vi "VelocityControl.vi"(0 "estimatives":T5, 1 "Dest_orientation":dbl, 2 "Position":dbl[](array[numeric]), 3 "Waypoint 1":dbl[](array[numeric]), 4 "Waypoint 0":dbl[](array[numeric]), 5 "Vx":dbl format="%#_13g", 7 "Project":T2, 9 "Vy":dbl format="%#_13g", 10 "VSSStates":T1, 11 "output xy":dbl=2.4, 12 "output inc":dbl=2.4, 13 "output angle":dbl=4.0, 14 "PID gains Vel":T4={"proportional gain (Kc)"=0.6, "integral time (Ti, min)"=0.0, "derivative time (Td, min)"=0.0}, 15 "Path  Smooth":dbl[][](array[numeric])) -> (8 "Output Velocity":dbl[](array[numeric]) format="%.2f")   [LabVIEW 2023]
uses:
  Controle/VelocityGraph.ctl
  Parameters_class/Project.ctl
  VSSNavigation/VSSAttackerStates.ctl
  <vilib>/Analysis/coordinate.llb/Wrap Angle (scalar).vi
  <vilib>/Analysis/coordinate.llb/2D Cartesian Coordinate Rotation (Scalar).vi
  <vilib>/Analysis/NI_AAL_Angle.lvlib
  <vilib>/Analysis/NI_AALPro.lvlib
panel:
  out "Velocity Y":T3
  out "Velocity X":T3
  in  "PID Gains Angle":T4={"proportional gain (Kc)"=5.0, "integral time (Ti, min)"=0.0, "derivative time (Td, min)"=-2.0}
  in  "Reinitialize":bool
  in  "PID Gains lateral":T4={"proportional gain (Kc)"=0.1, "integral time (Ti, min)"=0.0, "derivative time (Td, min)"=0.0}
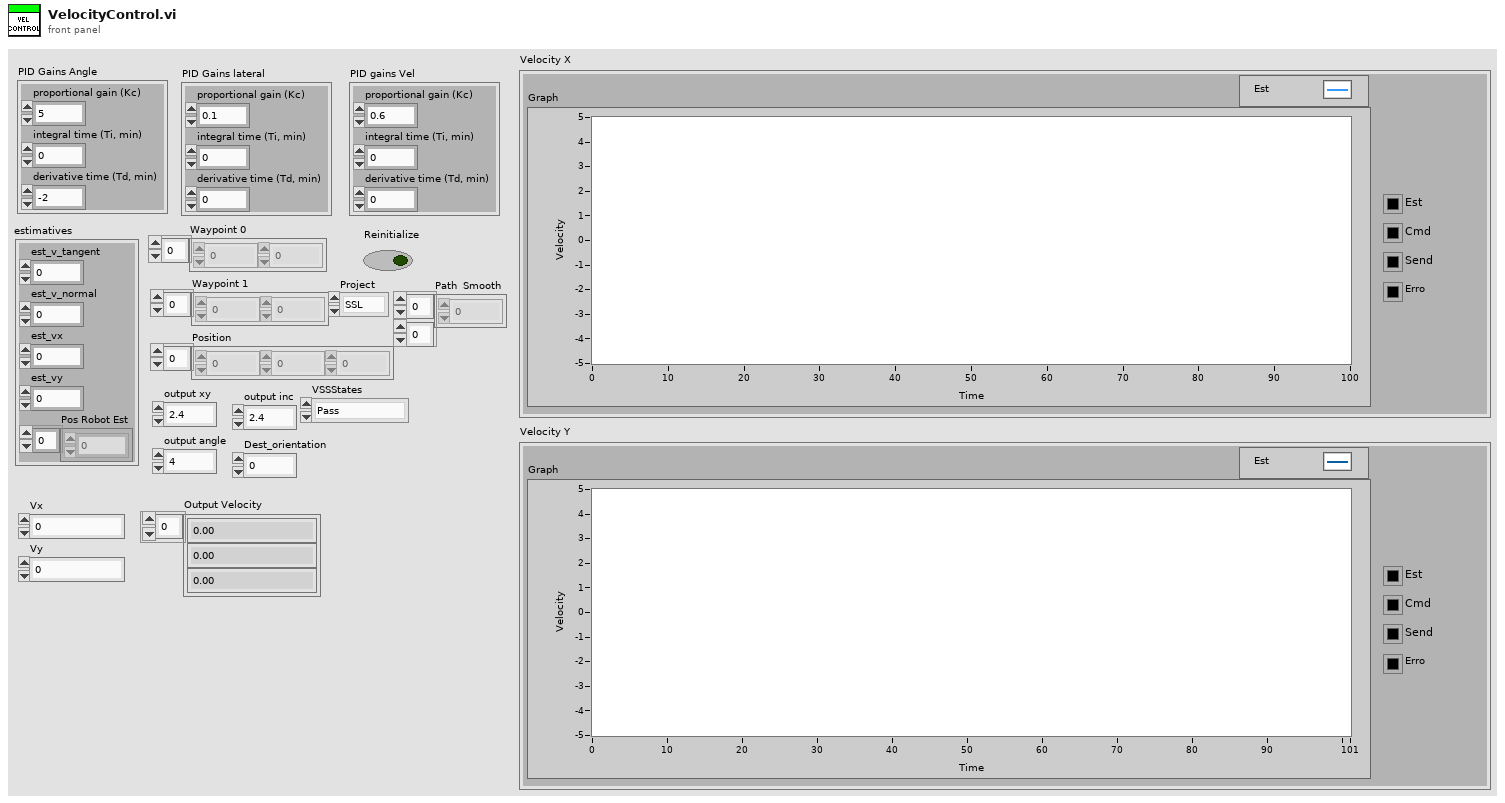
[diagram p1: front panel]
types:
  T1 = typedef "VSSAttackerStates.ctl" = enum16{"Pass", "GoToTangent", "BallGetting", "GoToKick", "Rotate anti-clockwise", "Rotate Clockwise", ""}
  T2 = typedef "Project.ctl" = enum16{"SSL", "VSS"}
  T3 = typedef "VelocityGraph.ctl" = cluster{"Graph":cluster{"est_vx":dbl, "Vx":dbl, dbl, "x out":dbl}, "Est":u32, "Cmd":u32, "Send":u32, "Erro":u32}
  T4 = cluster{"proportional gain (Kc)":dbl, "integral time (Ti, min)":dbl, "derivative time (Td, min)":dbl}
  T5 = cluster{"est_v_tangent":dbl, "est_v_normal":dbl, "est_vx":dbl, "est_vy":dbl, "Pos Robot Est":dbl[]}
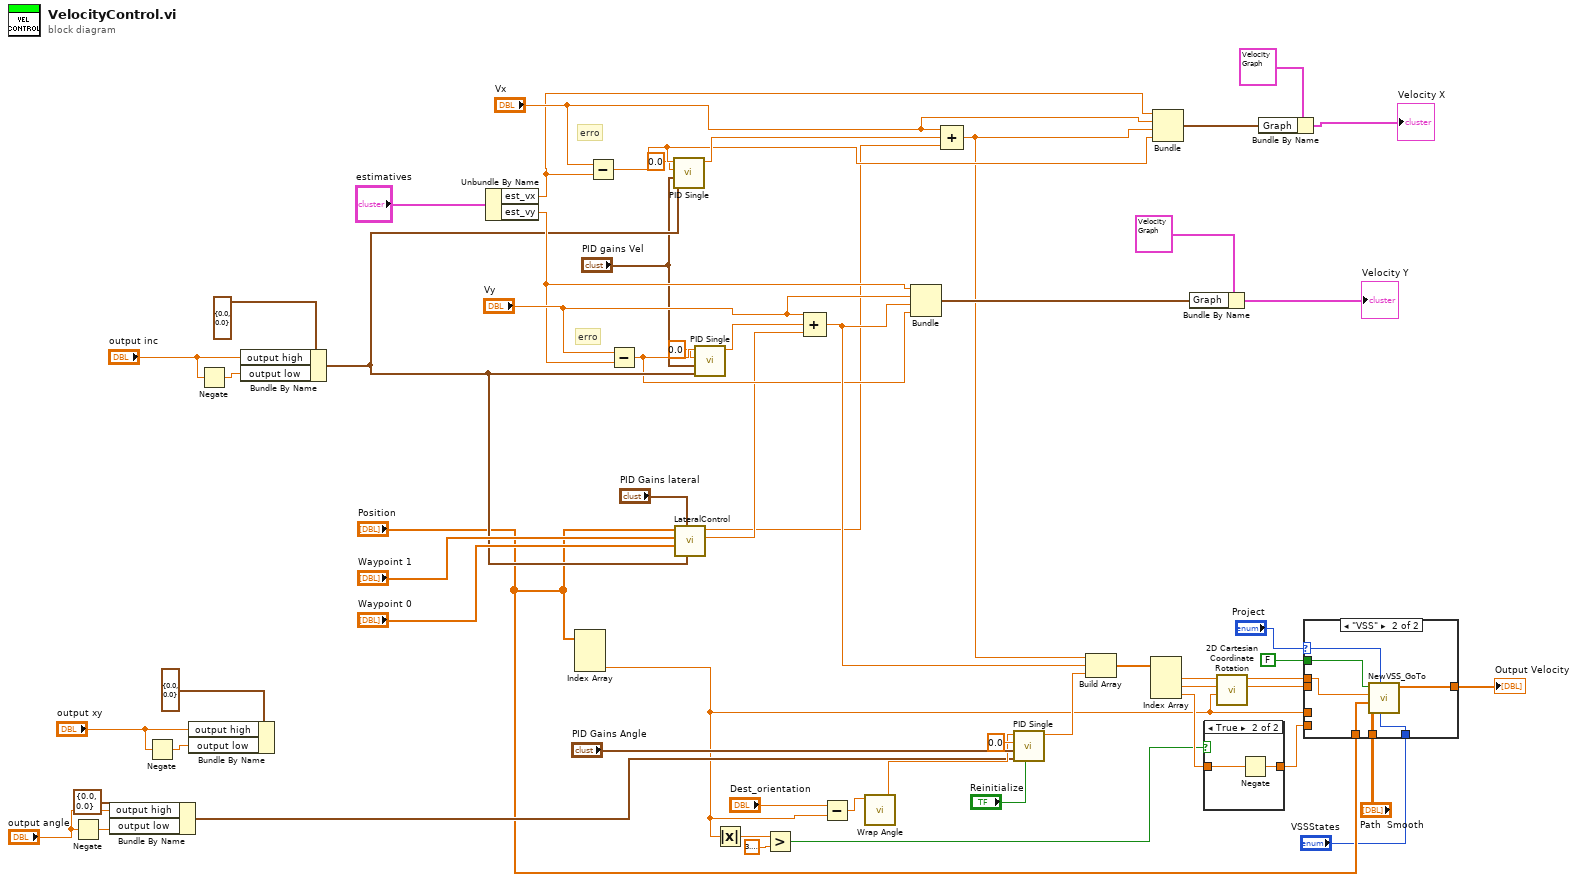
[diagram p0: block diagram]
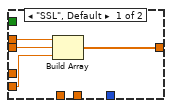
[diagram p2: hidden frame]
diagram:
  # "erro"
  # "erro"
  n1 = Negate(x="output angle") -> (-x=w43:dbl)
  n2 = Bundle By Name(cluster=cluster{"output high":dbl, "output low":dbl} {"output high"=0.0, "output low"=0.0}, "output high"="output angle", "output low"=w43) -> (w18:cluster{"output high":dbl, "output low":dbl})
  n3 = Negate(x="output xy") -> (-x=w45:dbl)
  n4 = Bundle By Name(cluster=cluster{"output high":dbl, "output low":dbl} {"output high"=0.0, "output low"=0.0} ("new element/subarray"), "output high"="output xy", "output low"=w45) -> ()  [unwired: 1 out]
  n5 = Negate(x="output inc") -> (-x=w28:dbl)
  n6 = Bundle By Name(cluster=cluster{"output high":dbl, "output low":dbl} {"output high"=0.0, "output low"=0.0} ("new element/subarray"), "output high"="output inc", "output low"=w28) -> (w17:cluster{"output high":dbl, "output low":dbl})
  n7 = Unbundle By Name("estimatives") -> ("est_vx"=w26:dbl, "est_vy"=w25:dbl)
  n8 = Index Array(array="Position") -> (element #3=w6:dbl)  [unwired: 3 in, 2 out]
  n9 = Subtract(x="Vx", y=w26) -> (x-y=w16:dbl)
  n10 = Subtract(x="Vy", y=w25) -> (x-y=w14:dbl)
  n11 = call "PID Single.vi"("Limits"=w17, "PID gains in"="PID gains Vel", "Variable"=0.0 ("Setpoint"), "Setpoint"=w16) -> ("Out"=w34:dbl)  [unwired: 7 in]
  n12 = call "LateralControl.vi"("output range"=w17, "PID Gains lateral"="PID Gains lateral", "Waypoint 0"="Waypoint 0", "Waypoint 1"="Waypoint 1", "Position"="Position") -> ("y out"=w11:dbl, "x out"=w10:dbl)  [unwired: 5 in]
  n13 = call "PID Single.vi"("Limits"=w17, "PID gains in"="PID gains Vel", "Variable"=0.0 ("Setpoint"), "Setpoint"=w14) -> ("Out"=w33:dbl)  [unwired: 7 in]
  n14 = Absolute Value(x=w6) -> (abs(x)=w57:dbl)
  n15 = Greater?(x=w57, y=3.141592653589793) -> (0:w52:bool)
  n16 = Compound Arithmetic op=ADD("Vy", w33, w11) -> (w30:dbl)
  n17 = Subtract(x="Dest_orientation", y=w6) -> (x-y=w49:dbl)
  n18 = call-poly <vilib>:"Wrap Angle.vi"("angle in"=w49) -> ("angle out"=w48:dbl)  [unwired: 9 in, 1 out]
  n19 = Bundle("est_vy"=w25, "Vy"="Vy", w30, w14) -> (w23:cluster{"est_vy":dbl, "Vy":dbl, dbl, dbl})  [unwired: 1 in]
  n20 = Compound Arithmetic op=ADD("Vx", w34, w10) -> (w9:dbl)
  n21 = call "PID Single.vi"("initialize"="Reinitialize", "Limits"=w18, "PID gains in"="PID Gains Angle", "Variable"=0.0, "Setpoint"=w48) -> ("Out"=w53:dbl)  [unwired: 6 in]
  n22 = Build Array(w9, w30, w53) -> (w7:dbl[])
  n23 = Index Array(array=w7) -> (element #1=w8:dbl, element #2=w60:dbl, element #3=w56:dbl)  [unwired: 3 in]
  n24 = Bundle("est_vx"=w26, "Vx"="Vx", w9, w16) -> (w20:cluster{"est_vx":dbl, "Vx":dbl, dbl, dbl})  [unwired: 1 in]
  n25 = Bundle By Name(cluster=T3 {"Graph"={"est_vx"=-0.14571416207204627, "Vx"=0.4692407651588243, 1.5797768746041183, "x out"=1.110536109445294}, "Est"=16860, "Cmd"=16711680, "Send"=6618880, "Erro"=16776722} ("Velocity Y"), "Graph"=w23) -> (→"Velocity Y":T3)
  n26 = case shown="True" w52 {
    tunnel: w56 -> [w61 w63]
    tunnel: [w61 w62] -> w55
    frame False {
    }
    frame True {
      n27 = Negate(x=w63) -> (-x=w62:dbl)
    }
  }
  n28 = call-poly <vilib>:"2D Cartesian Coordinate Rotation.vi"("theta"=w6, "y"=w60, "x"=w8) -> ("y out"=w58:dbl, "x out"=w59:dbl)  [unwired: 6 in, 1 out]
  n29 = Bundle By Name(cluster=T3 {"Graph"={"est_vx"=-0.14571416207204627, "Vx"=0.4692407651588243, 1.5797768746041183, "x out"=1.110536109445294}, "Est"=16860, "Cmd"=16711680, "Send"=6618880, "Erro"=16776722} ("Velocity Y"), "Graph"=w20) -> (→"Velocity X":T3)
  n30 = case shown="\"VSS\"" "Project" {
    selector: "Project" -> [_ w68]
    tunnel: w59 -> [w67 w73]
    tunnel: w58 -> [w66 _]
    tunnel: w55 -> [w65 _]
    tunnel: [w64 w74] -> w38
    tunnel: w6 -> [_ _]
    tunnel: "Path  Smooth" -> [_ w72]
    tunnel: FALSE -> [_ w71]
    tunnel: "Position" -> [_ w70]
    tunnel: "VSSStates" -> [_ w69]
    frame "SSL", Default {
      n31 = Build Array(w67, w66, w65) -> (w64:dbl[])
    }
    frame "VSS" {
      n32 = call "NewVSS_GoTo.vi"("VSSStates"=w69, "Numeric"=w68, "Path  Smooth"=w72, "Position"=w70, "V_tan(opitional)"=w73, "GoToNavigation?"=w71) -> ("Output Velocity"=w74:dbl[])  [unwired: 5 in]
    }
  }
  "Output Velocity" <- w38
